vi "calc pendulum params.vi"(3 "g":dbl=9.802, 4 "initialize":bool, 5 "m":dbl=0.5526, 6 "sample length":i32=10, 7 "z0":dbl=0.0492, 8 "energy calibration factor":dbl=1.0, 9 "pulse statistics":T3 {"timing error" format="%#.3p"}, 10 "ellipse fit":T1, 11 "crossing stats":T2) -> (0 "output cluster":T4, 1 "average pulse phase":dbl, 2 "average pulse energy":dbl format="%.2p")   [LabVIEW 2017]
uses:
  typedefs/crossing stats.ctl
  typedefs/magnetic field fit.ctl
  <vilib>/ptbypt/NI_PtbyPt.lvlib
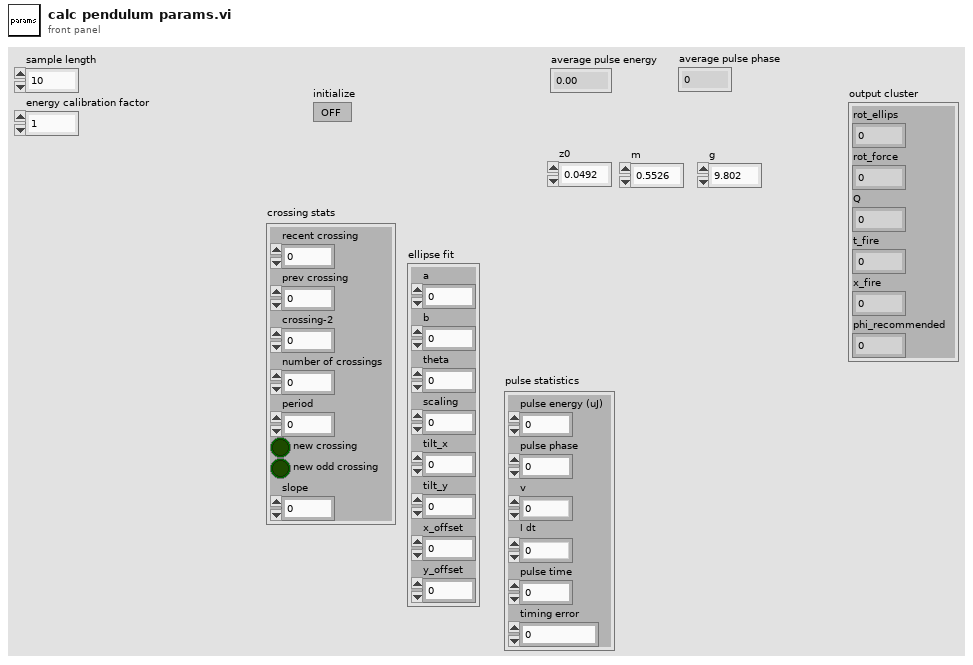
[diagram p1: front panel]
types:
  T1 = typedef "magnetic field fit.ctl" = cluster{"a":dbl, "b":dbl, "theta":dbl, "scaling":dbl, "tilt_x":dbl, "tilt_y":dbl, "bx_offset":dbl, "by_offset":dbl, "bz_offset":dbl, "x_offset":dbl, "y_offset":dbl}
  T2 = typedef "crossing stats.ctl" = cluster{"recent crossing":dbl, "prev crossing":dbl, "crossing-2":dbl, "number of crossings":i32, "period":dbl, "new crossing":bool, "new odd crossing":bool, "slope":dbl}
  T3 = cluster{"pulse energy (uJ)":sgl, "pulse phase":dbl, "v":dbl, "I dt":dbl, "pulse time":dbl, "timing error":dbl}
  T4 = cluster{"rot_ellips":dbl, "rot_force":dbl, "Q":dbl, "t_fire":dbl, "x_fire":dbl, "phi_recommended":dbl}
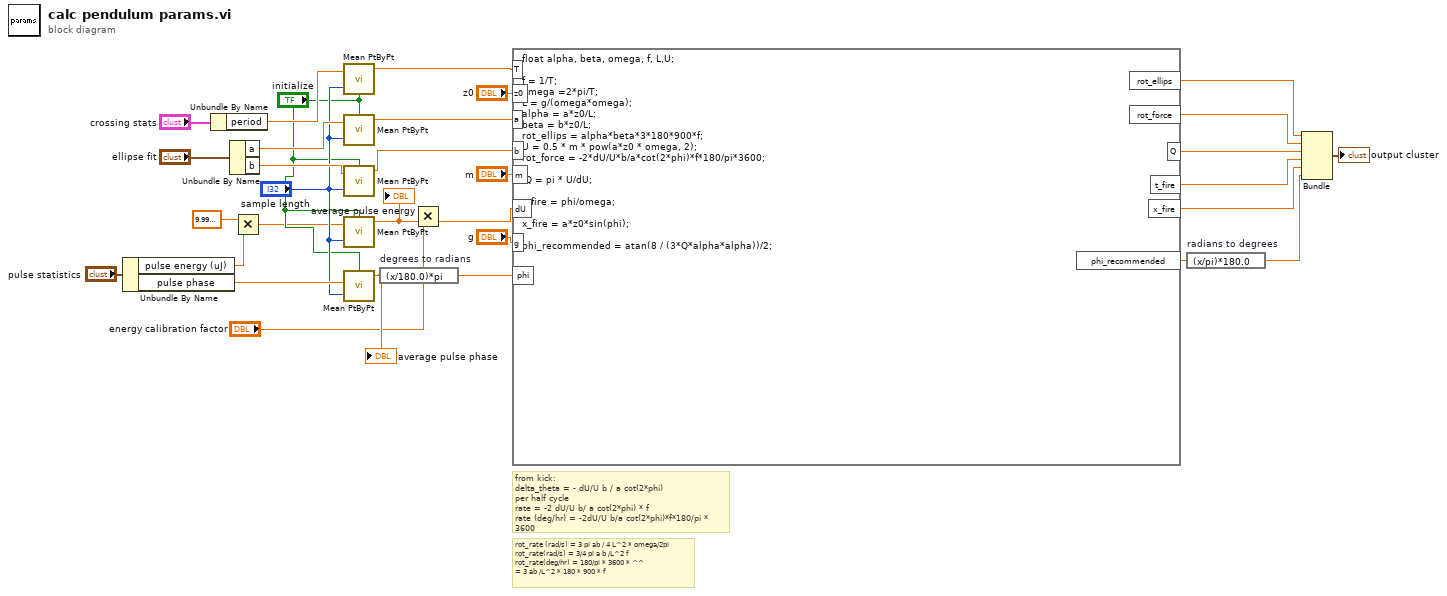
[diagram p0: block diagram]
diagram:
  # "from kick:\ndelta_theta = - dU/U b / a cot(2*phi)\nper half cycle\nrate = -2 dU/U b/ a cot(2*phi) * f\nrate (deg/hr) = -2dU/U b/a cot(2*phi)*f*180/pi * 3600"
  # "rot_rate (rad/s) = 3 pi ab / 4 L^2 * omega/2pi\nrot_rate(rad/s) = 3/4 pi a b /L^2 f\nrot_rate(deg/hr) = 180/pi * 3600 * ^^\n= 3 ab /L^2 * 180 * 900 * f"
  n1 = Unbundle By Name("pulse statistics") -> ("pulse energy (uJ)"=w25:sgl, "pulse phase"=w24:dbl)
  n2 = Unbundle By Name("crossing stats") -> ("period"=w30:dbl)
  n3 = Unbundle By Name("ellipse fit") -> ("a"=w28:dbl, "b"=w27:dbl)
  n4 = Multiply(x=sgl 1e-06, y=w25) -> (x*y=w6:sgl)
  n5 = call <vilib>:"Mean PtByPt.vi"("x"=w30, "sample length"="sample length", "initialize"="initialize") -> ("mean"=w13:dbl)  [unwired: 1 in, 1 out]
  n6 = call <vilib>:"Mean PtByPt.vi"("x"=w28, "sample length"="sample length", "initialize"="initialize") -> ("mean"=w12:dbl)  [unwired: 1 in, 1 out]
  n7 = call <vilib>:"Mean PtByPt.vi"("x"=w27, "sample length"="sample length", "initialize"="initialize") -> ("mean"=w11:dbl)  [unwired: 1 in, 1 out]
  n8 = call <vilib>:"Mean PtByPt.vi"("x"=w6, "sample length"="sample length", "initialize"="initialize") -> ("mean"=w9:dbl)  [unwired: 1 in, 1 out]
  "average pulse energy" <- w9
  n9 = call <vilib>:"Mean PtByPt.vi"("x"=w24, "sample length"="sample length", "initialize"="initialize") -> ("mean"=w3:dbl)  [unwired: 1 in, 1 out]
  "average pulse phase" <- w3
  n10 = expression code="(x/180.0)*pi" "degrees to radians"(w3) -> (w4:dbl)
  n11 = Multiply(x="energy calibration factor", y=w9) -> (x*y=w2:dbl)
  n12 = formula code="float alpha, beta, omega, f, L,U;\n\nf = 1/T;\nomega =2*pi/T;\nL = g/(omega*omega);\nalpha = a*z0/L;\nbeta = b*z0/L;\nrot_ellips = alpha*beta*3*180*900*f;\nU = 0.5 * m * pow(a*z0 * omega, 2);\nrot_force = -2*dU/U*b/a*cot(2*phi)*f*180/pi*3600;\n\n Q = pi * U/dU;\n\nt_fire = phi/omega;\n\nx_fire = a*z0*sin(phi);\n\nphi_recommended = atan(8 / (3*Q*alpha*alpha))/2;"("T"=w13, "z0"="z0", "a"=w12, "b"=w11, "m"="m", "dU"=w2, "g"="g", "phi"=w4) -> ("rot_ellips"=w20:dbl, "rot_force"=w19:dbl, "Q"=w18:dbl, "t_fire"=w17:dbl, "x_fire"=w16:dbl, "phi_recommended"=w15:dbl)
  n13 = expression code="(x/pi)*180.0" "radians to degrees"(w15) -> (w14:dbl)
  n14 = Bundle("rot_ellips"=w20, "rot_force"=w19, "Q"=w18, "t_fire"=w17, "x_fire"=w16, "phi_recommended"=w14) -> (→"output cluster":T4)  [unwired: 1 in]
